vi "补码转成十进制数1.vi"(11 "数组":bool[](array[boolean])) -> (3 "x+y 2":i16)   [LabVIEW 2012]
panel:
  out "非x?":bool[](array[boolean])
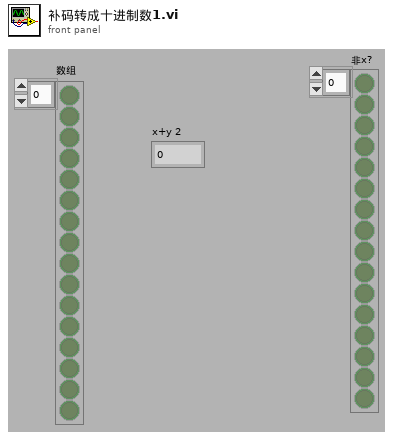
[diagram p1: front panel]
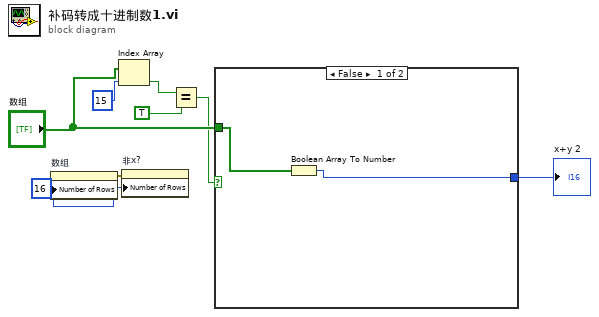
[diagram p0: block diagram]
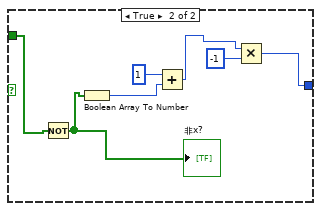
[diagram p2: hidden frame]
diagram:
  w1 = u32 16 ("行数")
  n1 = property on="数组" class="Arr (strict)"("Number of Rows"=w1) -> (error out=w2:errorcluster)  [unwired: 2 in, 1 out]
  n2 = Index Array(array="数组", index=15 ("索引")) -> (element=w6:bool)
  n3 = property on="非x?" class="Arr (strict)"(error in=w2, "Number of Rows"=w1) -> ()  [unwired: 1 in, 2 out]
  n4 = Equal?(x=w6, y=TRUE) -> (x = y?=w4:bool)
  n5 = case shown="False" w4 {
    tunnel: "数组" -> [w10 w14]
    tunnel: [w9 w11] -> w3
    frame False {
      n6 = Boolean Array To Number(Boolean array=w10) -> (number=w9:u32)
    }
    frame True {
      n7 = Not(x=w14) -> (.not. x?=w17:bool[])
      "非x?" <- w17
      n8 = Boolean Array To Number(Boolean array=w17) -> (number=w15:u32)
      n9 = Add(x=u32 1, y=w15) -> (x+y=w13:u32)
      n10 = Multiply(x=w13, y=-1) -> (x*y=w11:u32)
    }
  }
  "x+y 2" <- w3
